vi "Acquire and Log Data.vi"(0 "TDMS Refnum in":refnum<k34>, 1 "Simulate Data":bool, 5 "Refnum in":refnum<k20>[](array[refnum]), 7 "2 USRPs?":bool[](array[boolean]), 9 "Data Queue in":refnum<queue>, 11 "error in (no error)":errorcluster, 12 "Samples per Read":u32=1024000 format="%.3p", 13 "Previewed Channel":T1) -> (4 "TDMS Refnum out":refnum<k34>, 6 "Refnum out":refnum<k20>[](array[refnum]), 15 "error out":errorcluster)   [LabVIEW 2016]
uses:
  TDMS Raw to Channels/Previewed Channel - Enum.ctl
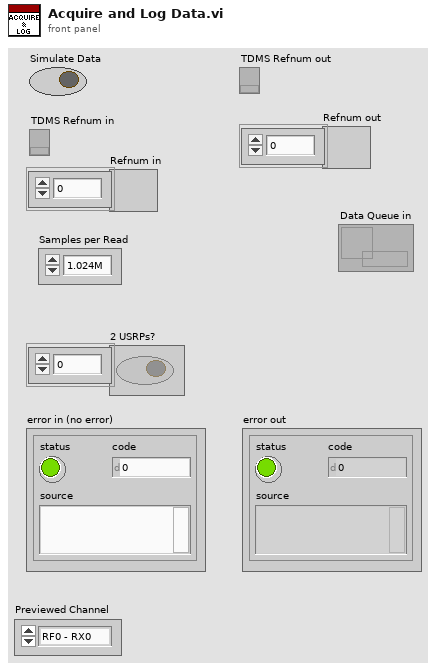
[diagram p1: front panel]
types:
  T1 = typedef "Previewed Channel - Enum.ctl" = enum16{"RF0 - RX0", "RF0 - RX1", "RF1 - RX0", "RF1 - RX1"}
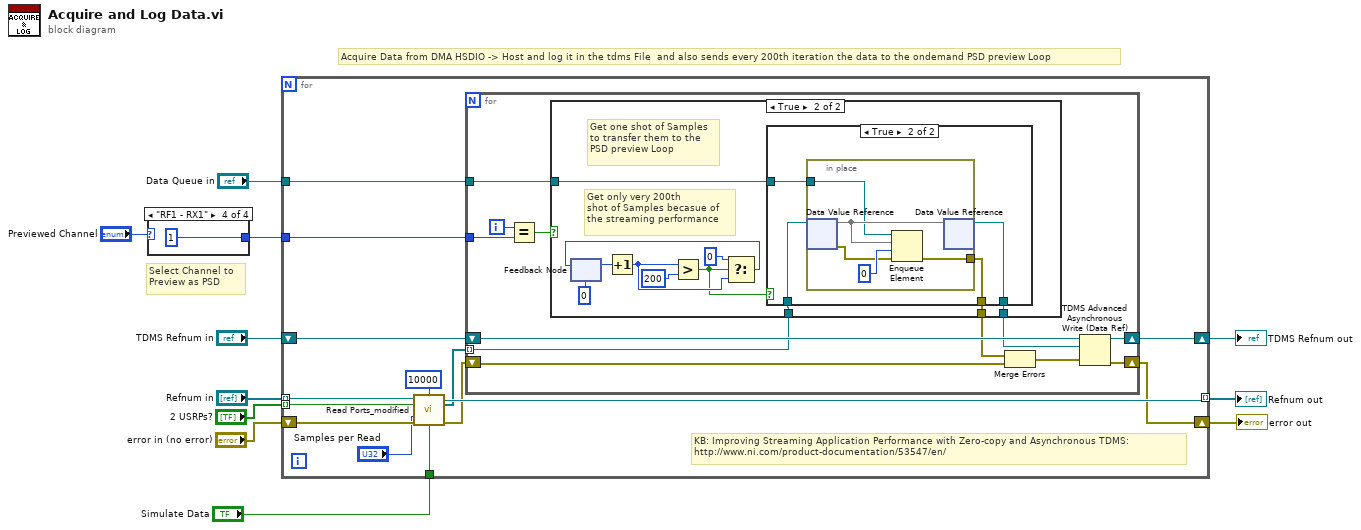
[diagram p0: block diagram]
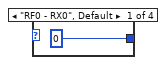
[diagram p2: hidden frame]
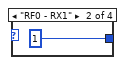
[diagram p3: hidden frame]
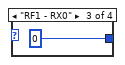
[diagram p4: hidden frame]
diagram:
  # "Select Channel to \nPreview as PSD"
  # "Acquire Data from DMA HSDIO -> Host and log it in the tdms File  and also sends every 200th iteration the data to the ondemand PSD preview Loop"
  n1 = case shown="\"RF1 - RX1\"" "Previewed Channel" {
    tunnel: [0 ("y") 1 ("y") 0 ("y") 1 ("y")] -> w1
    frame "RF0 - RX0", Default {
    }
    frame "RF0 - RX1" {
    }
    frame "RF1 - RX0" {
    }
    frame "RF1 - RX1" {
    }
  }
  n2 = for {
    tunnel: "Refnum in" -> [w28] mode=indexing
    shift-right: [w18] -> w9
    shift-left: "error in (no error)" -> [w29]
    tunnel: "2 USRPs?" -> [w25] mode=indexing
    tunnel: [w24] -> w5 mode=indexing
    tunnel: "Simulate Data" -> [w26]
    shift-right: [w21] -> w11
    shift-left: "TDMS Refnum in" -> [w22]
    tunnel: "Data Queue in" -> [w17]
    tunnel: w1 -> [w16]
    # "KB: Improving Streaming Application Performance with Zero-copy and Asynchronous TDMS:\nhttp://www.ni.com/product-documentation/53547/en/"
    n3 = call "Read Ports_modified.vi"("Refnum in"=w28, "timeout (ms)"=10000 ("Timeout (ms)"), "All 4 Ports"=w25, "number of elements"="Samples per Read", "error in"=w29, "Simulated Data"=w26) -> ("Refnum out"=w24:refnum<k20>, "Read Region References"=w20:refnum<data-value>[], "error out"=w19:errorcluster)  [unwired: 4 in, 3 out]
    n4 = for {
      shift-right: [w40] -> w21
      shift-left: w22 -> [w41]
      tunnel: w20 -> [w37] mode=indexing
      shift-right: [w39] -> w18
      shift-left: w19 -> [w31]
      tunnel: w17 -> [w38]
      tunnel: w16 -> [w33]
      i -> [w35]
      n5 = Equal?(x=w35, y=w33) -> (x = y?=w34:bool)
      n6 = case shown="True" w34 {
        tunnel: w38 -> [_ w53]
        tunnel: w37 -> [w42 w52]
        tunnel: [w42 w51] -> w36
        tunnel: [_ w43] -> w30
        frame False {
        }
        frame True {
          # "Get only very 200th \nshot of Samples becasue of \nthe streaming performance"
          # "Get one shot of Samples\nto transfer them to the \nPSD preview Loop"
          n7 = feedback #1(u32 0 ("y")) -> (w50:u32)
          n8 = Increment(x=w50) -> (x+1=w46:u32)
          n9 = Greater?(x=w46, y=u32 200) -> (0:w45:bool)
          n10 = Select(t=u32 0 ("y"), s=w45, f=w46) -> (s? t:f=w44:u32)
          n11 = feedback-in #1(w44) -> ()
          n12 = case shown="True" w45 {
            tunnel: w53 -> [_ w58]
            tunnel: w52 -> [w54 w57]
            tunnel: [w54 w56] -> w51
            tunnel: [_ w55] -> w43
            frame False {
            }
            frame True {
              n13 = in-place {
                in-place-border: w58 -> [w62]
                in-place-border: [w59] -> w55
                n14 = in-place-dvr #2(w57) -> (w63:u64[], w60:errorcluster)
                n15 = Enqueue Element(queue=w62, element=w63, timeout in ms (-1)=0, error in (no error)=w60) -> (error out=w59:errorcluster)  [unwired: 2 out]
                n16 = in-place-dvr #2(w63) -> (w56:refnum<data-value>)  [unwired: 1 out]
              }
            }
          }
        }
      }
      n17 = Merge Errors(w30, w31) -> (w32:errorcluster)
      n18 = TDMS Advanced Asynchronous Write (Data Ref)(8:w32, 10:w36, 11:w41) -> (0:w39:errorcluster, 3:w40:refnum<k34>)  [unwired: 1 in]
    }
  }
  "TDMS Refnum out" <- w11
  "error out" <- w9
  "Refnum out" <- w5
